vi "Expand-Shrink Front Panel Right.vi"(6 "Side Panel Size":i32=320, 8 "Error In":errorcluster, 10 "Expand(T)/Shrink":bool=TRUE, 11 "VI Refnum":refnum<vi>) -> (0 "Error Out":errorcluster)   [LabVIEW 2021, in "GUI.lvlib"]
uses:
  GUI.lvlib
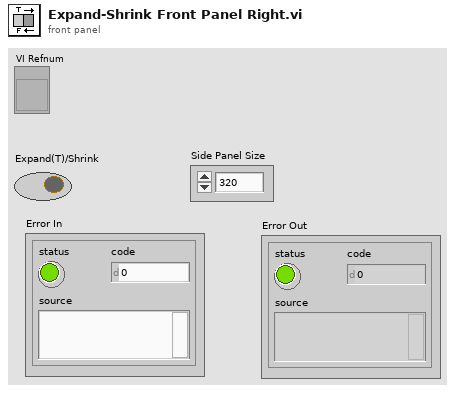
[diagram p1: front panel]
types:
  T1 = typedef "LVRectTypeDef.ctl" = cluster{"Left":i16, "Top":i16, "Right":i16, "Bottom":i16}
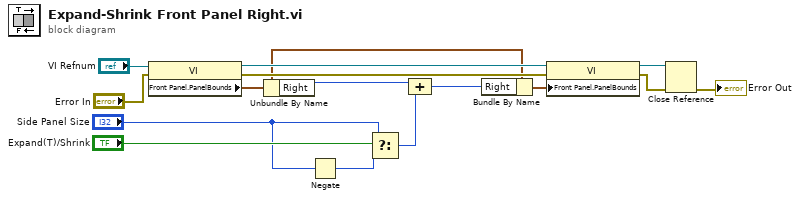
[diagram p0: block diagram]
diagram:
  n1 = property class="VI"(reference="VI Refnum", error in="Error In") -> (reference out=w13:refnum<vi>, error out=w12:errorcluster, "Front Panel.PanelBounds"=w10:T1)
  n2 = Unbundle By Name(w10) -> ("Right"=w14:i16)
  n3 = Negate(x="Side Panel Size") -> (-x=w1:i32)
  n4 = Select(t="Side Panel Size", s="Expand(T)/Shrink", f=w1) -> (s? t:f=w3:i32)
  n5 = Compound Arithmetic op=ADD(w14, w3) -> (w8:i32)
  n6 = Bundle By Name(cluster=w10, "Right"=w8) -> (w9:T1)
  n7 = property class="VI"(reference=w13, error in=w12, "Front Panel.PanelBounds"=w9) -> (reference out=w11:refnum<vi>, error out=w6:errorcluster)
  n8 = Close Reference(reference=w11, error in (no error)=w6) -> (error out=→"Error Out":errorcluster)
